vi "propnodotnet.vi"   [LabVIEW 2014]
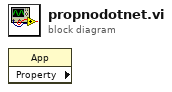
[diagram p0: block diagram]
diagram:
  n1 = property class="App" props=[]() -> ()  [unwired: 2 in, 3 out]
